vi "set_centering.vi"(0 "TrajectoryTS090820Circular2D in":refnum<class "TrajectoryTS090820Circular2D.lvclass">, 1 "x center":dbl, 2 "y center":dbl, 3 "z center":dbl, 4 "rotation angle":dbl, 5 "error in (no error)":errorcluster) -> (14 "TrajectoryTS090820Circular2D out":refnum<class "TrajectoryTS090820Circular2D.lvclass">, 19 "error out":errorcluster)   [LabVIEW 2010, in "TrajectoryTS090820Circular2D.lvclass"]
uses:
  TrajectoryTS090820Circular2D.lvclass
  TrajectoryTS090820Circular2D.lvclass/TrajectoryTS090820Circular2D.ctl
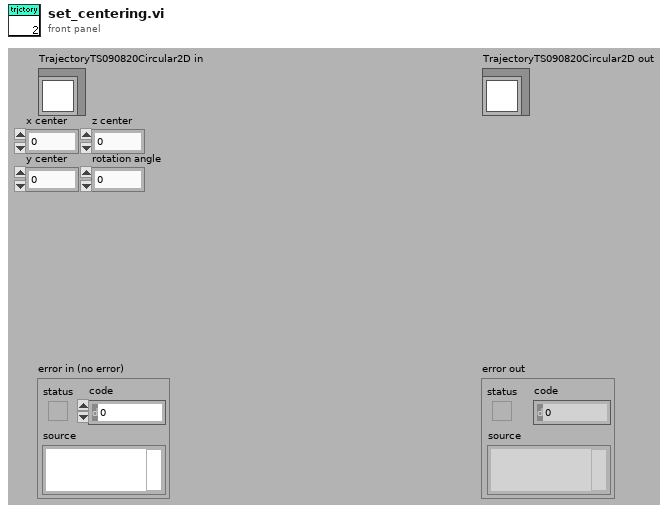
[diagram p1: front panel]
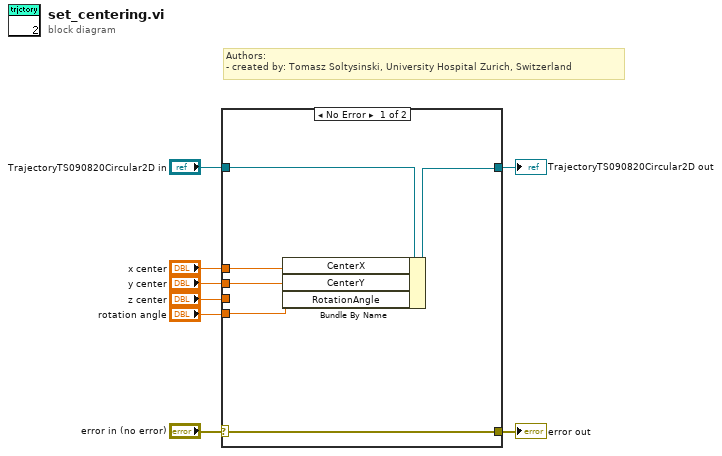
[diagram p0: block diagram]
diagram:
  # "Authors: \n- created by: Tomasz Soltysinski, University Hospital Zurich, Switzerland"
  n1 = case shown="No Error" "error in (no error)" {
    selector: "error in (no error)" -> [w14 w16]
    tunnel: [w14 w16] -> w7
    tunnel: [w12 w15] -> w5
    tunnel: "TrajectoryTS090820Circular2D in" -> [w13 w15]
    tunnel: "x center" -> [w11 _]
    tunnel: "y center" -> [w10 _]
    tunnel: "z center" -> [_ _]
    tunnel: "rotation angle" -> [w9 _]
    frame No Error {
      n2 = Bundle By Name(cluster=w13, "CenterX"=w11, "CenterY"=w10, "RotationAngle"=w9) -> (w12:refnum<class "TrajectoryTS090820Circular2D.lvclass">)
    }
    frame Error {
    }
  }
  "error out" <- w7
  "TrajectoryTS090820Circular2D out" <- w5
